vi "extractText.vi"(8 "error in (no error)":errorcluster, 11 "xwpfWriter in":refnum<class "xwpfWriter.lvclass">) -> (0 "error out":errorcluster, 2 "Text":string, 3 "xwpfWriter out":refnum<class "xwpfWriter.lvclass">)   [LabVIEW 2017, in "LabVIEW NPOI.lvlib" / "xwpfWriter.lvclass"]
uses:
  xwpfWriter.lvclass
  xwpfWriter.lvclass/xwpfWriter.ctl
  C:/Users/Neo/Desktop/Dev_Tools_BR/LabVIEW_NPOI/lib/NPOI 2.1.1/NPOI.OOXML.dll
  lib/NPOI 2.1.1/NPOI.OOXML.dll
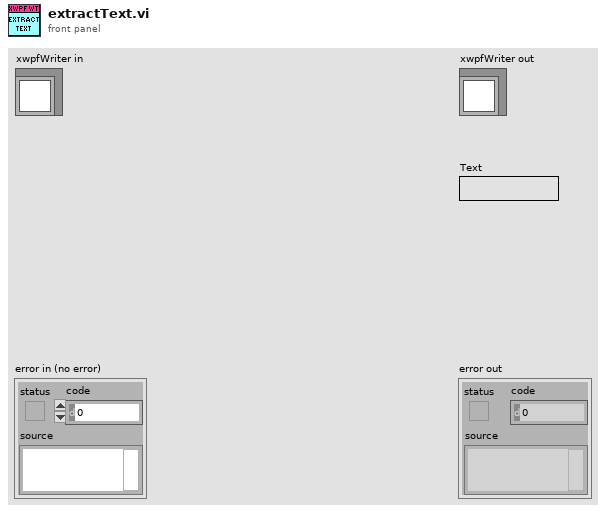
[diagram p1: front panel]
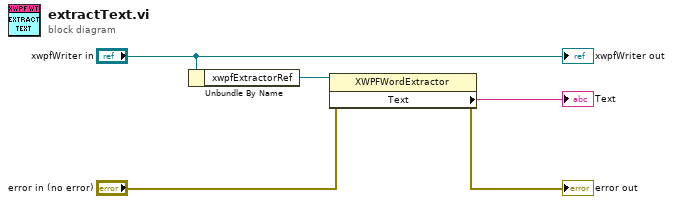
[diagram p0: block diagram]
diagram:
  n1 = Unbundle By Name("xwpfWriter in") -> ("xwpfExtractorRef"=w4:refnum<k24>)
  n2 = property class="XWPFWordExtractor"(reference=w4, error in="error in (no error)") -> (error out=→"error out":errorcluster, "Text"=→"Text":string)  [unwired: 1 out]
  "xwpfWriter out" <- "xwpfWriter in"
